vi "加标回收启动对话框.vi"(11 "测试模式":enum16{"水样测试", "平行样测试", "加标回收", "集成干预测试"}(ring)) -> (1 "流程参数":T1, 2 "启动参数":T2, 3 "check ？":bool)   [LabVIEW 2016, in "质控单元V1.lvlib"]
panel:
  in  "采配水":bool=TRUE
  in  "取消":bool
  in  "确认":bool
  in  "CODCr":bool caption="启用"
  in  "CODMn":bool caption="启用"
  in  "总氮":bool caption="启用"
  in  "总磷":bool caption="启用"
  in  "氨氮":bool caption="启用"
  # "请选择启动参数和流程"
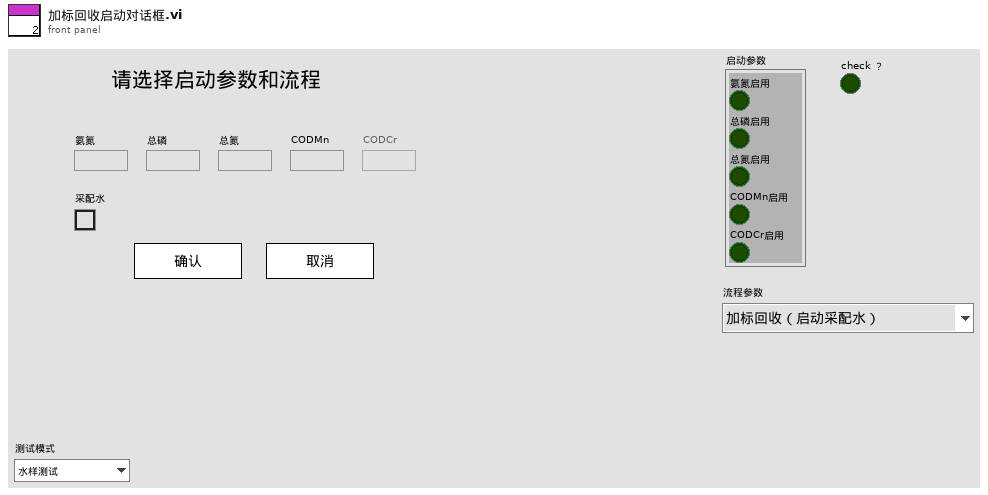
[diagram p1: front panel]
types:
  T1 = typedef "质控单元V1.lvlib/测试流程.ctl" = enum16{"加标回收（启动采配水）", "加标回收（不启动采配水）", "水样测试（启动采配水）", "水样测试（不启动采配水）", "平行样测试（启动采配水）", "平行样测试（不启动采配水）", "集成干预测试"}
  T2 = cluster{"氨氮启用":bool, "总磷启用":bool, "总氮启用":bool, "CODMn启用":bool, "CODCr启用":bool}
  T3 = cluster{"氨氮":bool, "总磷":bool, "总氮":bool, "CODMn":bool, "CODCr":bool, "氨氮总磷":bool, "总磷总氮":bool}
  T4 = cluster{"氨氮":bool, "总磷":bool, "总氮":bool, "CODMn":bool, "CODCr":bool}
  T5 = enum8{"Enabled", "Disabled", "Disabled and Grayed Out"}
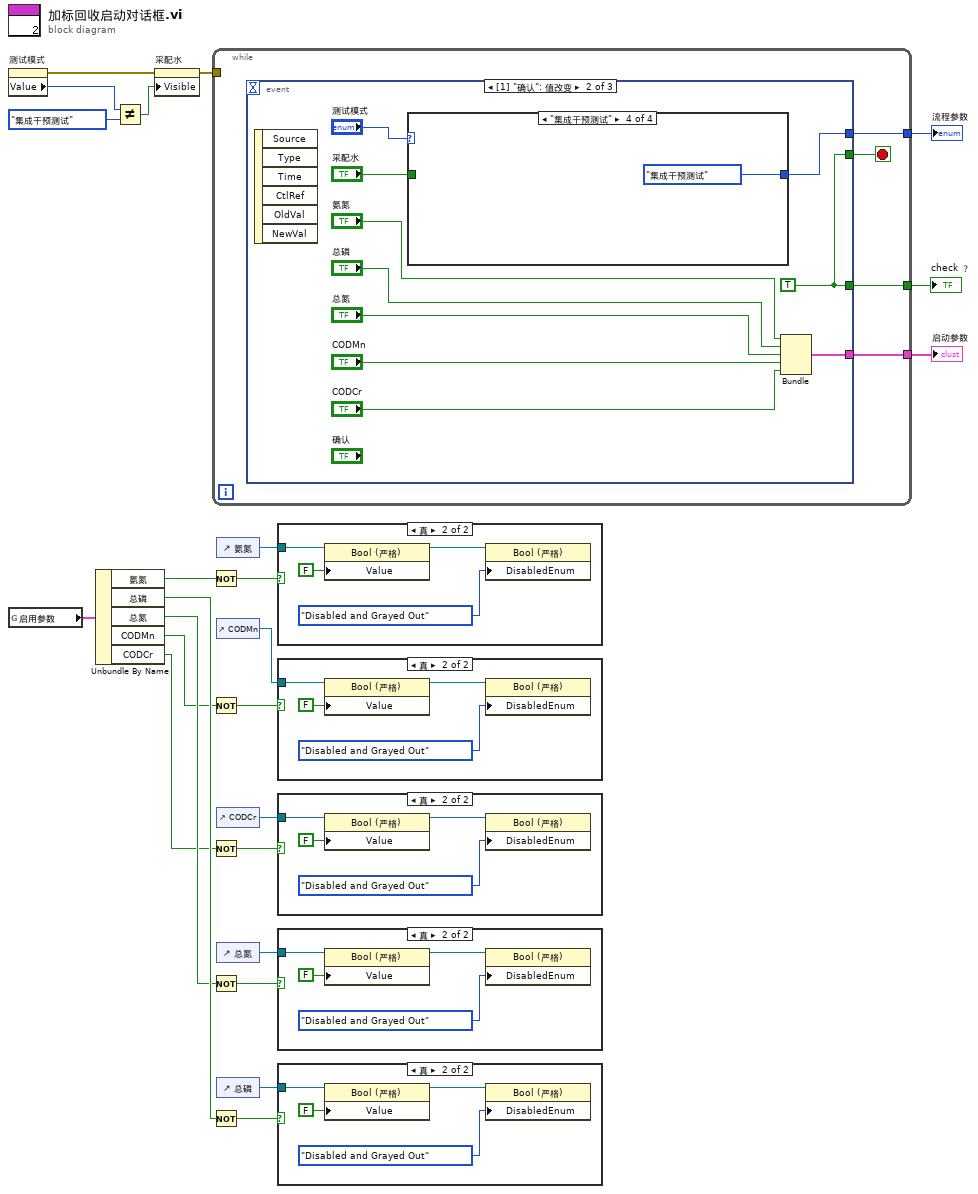
[diagram p0: block diagram]
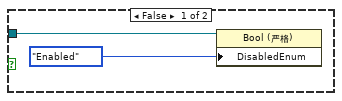
[diagram p2: hidden frame]
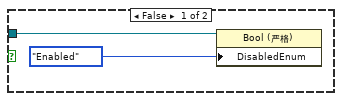
[diagram p3: hidden frame]
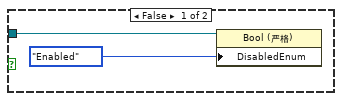
[diagram p4: hidden frame]
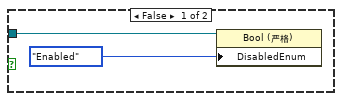
[diagram p5: hidden frame]
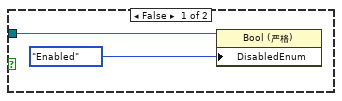
[diagram p6: hidden frame]
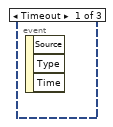
[diagram p7: hidden frame]
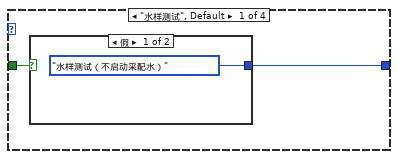
[diagram p8: hidden frame]
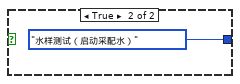
[diagram p9: hidden frame]
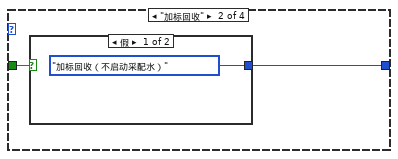
[diagram p10: hidden frame]
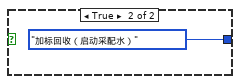
[diagram p11: hidden frame]
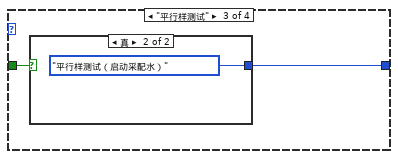
[diagram p12: hidden frame]
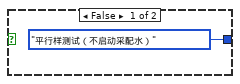
[diagram p13: hidden frame]
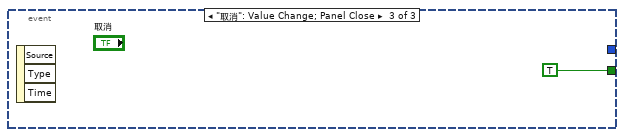
[diagram p14: hidden frame]
diagram:
  n1 = property on="测试模式" class="Enum (严格)"() -> (error out=w8:errorcluster, "Value"=w10:enum16{"水样测试", "平行样测试", "加标回收", "集成干预测试"})  [unwired: 2 in, 1 out]
  n2 = global read "ZK断电保存全局变量.vi" "启用参数"() -> (w16:T3)
  n3 = Unbundle By Name(w16) -> ("氨氮"=w14:bool, "总磷"=w15:bool, "总氮"=w13:bool, "CODMn"=w12:bool, "CODCr"=w11:bool)
  n4 = Not Equal?(x=w10, y=enum16{"水样测试", "平行样测试", "加标回收", "集成干预测试"}."集成干预测试") -> (x != y?=w7:bool)
  n5 = property on="采配水" class="Bool (严格)"(error in=w8, "Visible"=w7) -> (error out=w6:errorcluster)  [unwired: 1 in, 1 out]
  n6 = Not(x=w14) -> (.not. x?=w2:bool)
  n7 = Not(x=w12) -> (.not. x?=w5:bool)
  n8 = Not(x=w11) -> (.not. x?=w4:bool)
  n9 = Not(x=w13) -> (.not. x?=w3:bool)
  n10 = Not(x=w15) -> (.not. x?=w1:bool)
  n11 = while {
    tunnel: [w28] -> w24
    tunnel: [w26] -> w23
    tunnel: [w25] -> w22
    tunnel: w6 -> [_]
    stop <- w27 stop-if-true
    n12 = event shown="[1] \"确认\": 值改变" {
      selector: _ -> [_ _ _]
      dyn-events: _ -> [_ _ _]
      timeout: _ -> [_ _ _]
      tunnel: [_ w38 _] -> w28
      tunnel: [_ w38 TRUE] -> w27
      tunnel: [_ w32 _] -> w26
      tunnel: [_ w30 _] -> w25
      event Timeout {
        n13 = event-data() -> ()  [unwired: 1 in, 3 out]
      }
      event "确认": Value Change {
        w38 = TRUE
        n14 = event-data() -> ()  [unwired: 1 in, 6 out]
        n15 = case shown="\"集成干预测试\"" "测试模式" {
          tunnel: "采配水" -> [w40 w44 w48 _]
          tunnel: [w39 w43 w47 测试流程."集成干预测试" ("流程")] -> w30
          frame "水样测试", Default {
            n16 = case shown="假" w40 {
              tunnel: [测试流程."水样测试（不启动采配水）" ("流程") 测试流程."水样测试（启动采配水）" ("流程")] -> w39
              frame False {
              }
              frame True {
              }
            }
          }
          frame "加标回收" {
            n17 = case shown="假" w44 {
              tunnel: [测试流程."加标回收（不启动采配水）" ("流程") 测试流程."加标回收（启动采配水）" ("流程")] -> w43
              frame False {
              }
              frame True {
              }
            }
          }
          frame "平行样测试" {
            n18 = case shown="真" w48 {
              tunnel: [测试流程."平行样测试（不启动采配水）" ("流程") 测试流程."平行样测试（启动采配水）" ("流程")] -> w47
              frame False {
              }
              frame True {
              }
            }
          }
          frame "集成干预测试" {
          }
        }
        n19 = Bundle("氨氮"="氨氮", "总磷"="总磷", "总氮"="总氮", "CODMn"="CODMn", "CODCr"="CODCr") -> (w32:T4)  [unwired: 1 in]
      }
      event "取消": Value Change; Panel Close {
        n20 = event-data() -> ()  [unwired: 1 in, 3 out]
      }
    }
  }
  "check ？" <- w24
  "启动参数" <- w23
  "流程参数" <- w22
  n21 = control-ref of="氨氮"() -> (w21:refnum<vi>)
  n22 = control-ref of="CODMn"() -> (w18:refnum<vi>)
  n23 = control-ref of="CODCr"() -> (w17:refnum<vi>)
  n24 = control-ref of="总氮"() -> (w19:refnum<vi>)
  n25 = control-ref of="总磷"() -> (w20:refnum<vi>)
  n26 = case shown="真" w2 {
    tunnel: w21 -> [w53 w58]
    frame False {
      n27 = property class="Bool (严格)"(reference=w53, "DisabledEnum"=T5."Enabled" ("禁用")) -> ()  [unwired: 1 in, 2 out]
    }
    frame True {
      n28 = property class="Bool (严格)"(reference=w58, "Value"=FALSE ("值")) -> (reference out=w56:refnum<vi>)  [unwired: 1 in, 1 out]
      n29 = property class="Bool (严格)"(reference=w56, "DisabledEnum"=T5."Disabled and Grayed Out" ("禁用")) -> ()  [unwired: 1 in, 2 out]
    }
  }
  n30 = case shown="真" w5 {
    tunnel: w18 -> [w59 w64]
    frame False {
      n31 = property class="Bool (严格)"(reference=w59, "DisabledEnum"=T5."Enabled" ("禁用")) -> ()  [unwired: 1 in, 2 out]
    }
    frame True {
      n32 = property class="Bool (严格)"(reference=w64, "Value"=FALSE ("值")) -> (reference out=w62:refnum<vi>)  [unwired: 1 in, 1 out]
      n33 = property class="Bool (严格)"(reference=w62, "DisabledEnum"=T5."Disabled and Grayed Out" ("禁用")) -> ()  [unwired: 1 in, 2 out]
    }
  }
  n34 = case shown="真" w4 {
    tunnel: w17 -> [w65 w70]
    frame False {
      n35 = property class="Bool (严格)"(reference=w65, "DisabledEnum"=T5."Enabled" ("禁用")) -> ()  [unwired: 1 in, 2 out]
    }
    frame True {
      n36 = property class="Bool (严格)"(reference=w70, "Value"=FALSE ("值")) -> (reference out=w68:refnum<vi>)  [unwired: 1 in, 1 out]
      n37 = property class="Bool (严格)"(reference=w68, "DisabledEnum"=T5."Disabled and Grayed Out" ("禁用")) -> ()  [unwired: 1 in, 2 out]
    }
  }
  n38 = case shown="真" w3 {
    tunnel: w19 -> [w71 w76]
    frame False {
      n39 = property class="Bool (严格)"(reference=w71, "DisabledEnum"=T5."Enabled" ("禁用")) -> ()  [unwired: 1 in, 2 out]
    }
    frame True {
      n40 = property class="Bool (严格)"(reference=w76, "Value"=FALSE ("值")) -> (reference out=w74:refnum<vi>)  [unwired: 1 in, 1 out]
      n41 = property class="Bool (严格)"(reference=w74, "DisabledEnum"=T5."Disabled and Grayed Out" ("禁用")) -> ()  [unwired: 1 in, 2 out]
    }
  }
  n42 = case shown="真" w1 {
    tunnel: w20 -> [w77 w82]
    frame False {
      n43 = property class="Bool (严格)"(reference=w77, "DisabledEnum"=T5."Enabled" ("禁用")) -> ()  [unwired: 1 in, 2 out]
    }
    frame True {
      n44 = property class="Bool (严格)"(reference=w82, "Value"=FALSE ("值")) -> (reference out=w80:refnum<vi>)  [unwired: 1 in, 1 out]
      n45 = property class="Bool (严格)"(reference=w80, "DisabledEnum"=T5."Disabled and Grayed Out" ("禁用")) -> ()  [unwired: 1 in, 2 out]
    }
  }
